vi "TCP Read with Size.vi"(8 "error in (no error)":errorcluster, 9 "timeout ms (25000)":i32=25000, 11 "connection ID":refnum<k5>) -> (0 "error out":errorcluster, 2 "data out":string, 3 "connection ID out":refnum<k5>)   [LabVIEW 2015]
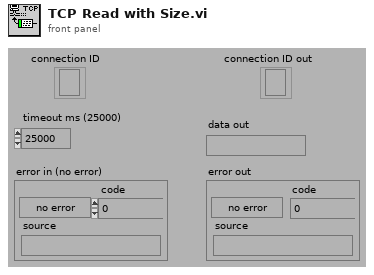
[diagram p1: front panel]
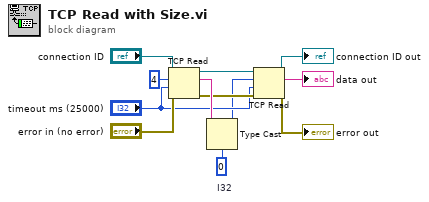
[diagram p0: block diagram]
diagram:
  w8 = 0  # I32
  n1 = TCP Read(connection ID="connection ID", bytes to read=4, error in (no error)="error in (no error)", 9:"timeout ms (25000)") -> (connection ID out=w7:refnum<k5>, data out=w9:string, error out=w6:errorcluster)  [unwired: 1 in]
  n2 = Type Cast(type=w8, x=w9) -> (*(type *) &x=w1:i32)
  n3 = TCP Read(connection ID=w7, bytes to read=w1, error in (no error)=w6, 9:"timeout ms (25000)") -> (connection ID out=→"connection ID out":refnum<k5>, data out=→"data out":string, error out=→"error out":errorcluster)  [unwired: 1 in]
